vi "Get SplitMode.vi"(8 "error in (no error)":errorcluster caption="错误输入（无错误）", 11 "PanelDataNode 输入":refnum<class "PanelDataNode.lvclass"> caption="DNL_LabVIEW Object in") -> (0 "error out":errorcluster caption="错误输出", 2 "Split Mode":i32, 3 "PanelDataNode 输出":refnum<class "PanelDataNode.lvclass"> caption="DNL_LabVIEW Object out")   [LabVIEW 2016, in "PanelDataNode.lvclass"]
uses:
  PanelDataNode.lvclass
  PanelDataNode.lvclass/PanelDataNode.ctl
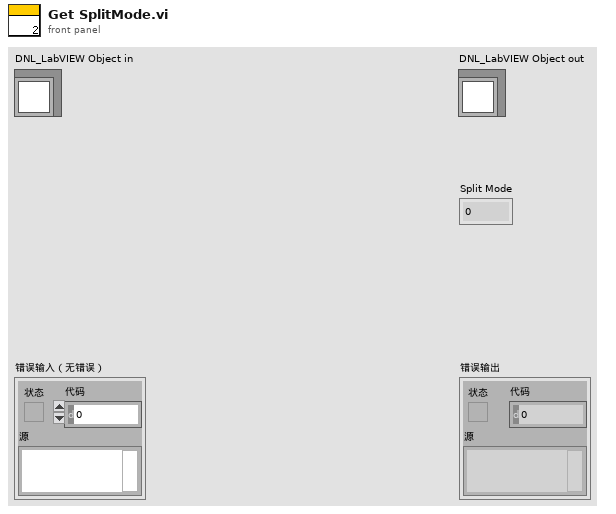
[diagram p1: front panel]
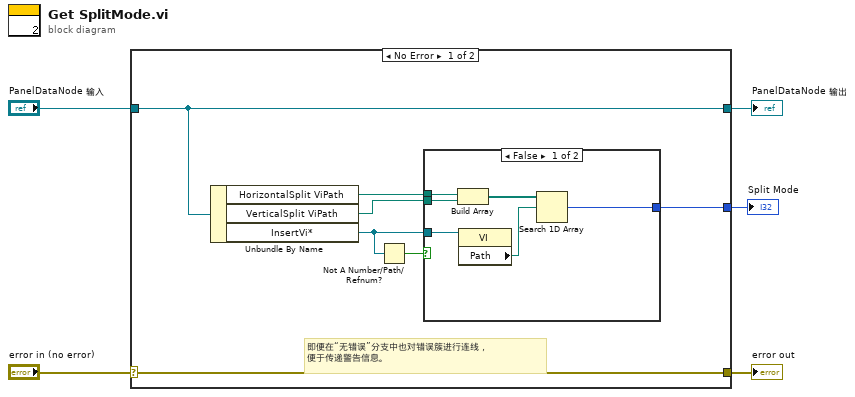
[diagram p0: block diagram]
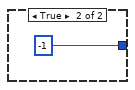
[diagram p2: hidden frame]
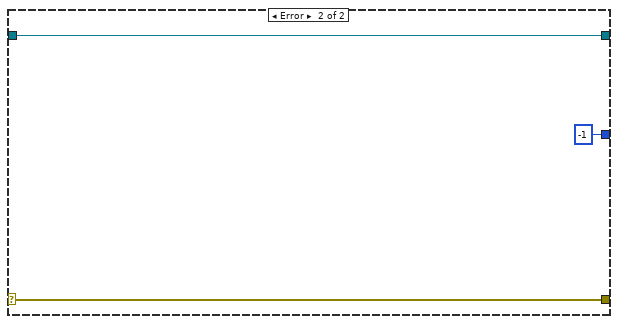
[diagram p3: hidden frame]
diagram:
  n1 = case shown="No Error" "error in (no error)" {
    selector: "error in (no error)" -> [w12 w22]
    tunnel: [w12 w22] -> w4
    tunnel: [w11 w21] -> w2
    tunnel: "PanelDataNode 输入" -> [w11 w21]
    tunnel: [w6 -1 ("index of element")] -> w1
    frame No Error {
      # "即便在“无错误”分支中也对错误簇进行连线，\n便于传递警告信息。"
      n2 = Unbundle By Name(w11) -> ("HorizontalSplit ViPath"=w10:path, "VerticalSplit ViPath"=w9:path, "InsertVi*"=w7:refnum<vi>)
      n3 = Not A Number/Path/Refnum?(number/path/refnum=w7) -> (NaN/Path/Refnum?=w8:bool)
      n4 = case shown="False" w8 {
        tunnel: w10 -> [w18 _]
        tunnel: w9 -> [w17 _]
        tunnel: w7 -> [w14 _]
        tunnel: [w13 -1 ("index of element")] -> w6
        frame False {
          n5 = Build Array(w18, w17) -> (w16:path[])
          n6 = property class="VI"(reference=w14) -> ("Path"=w15:path)  [unwired: 1 in, 2 out]
          n7 = Search 1D Array(1D array=w16, element=w15) -> (index of element=w13:i32)  [unwired: 1 in]
        }
        frame True {
        }
      }
    }
    frame Error {
    }
  }
  "error out" <- w4
  "PanelDataNode 输出" <- w2
  "Split Mode" <- w1
